vi "Sample mono.vi"() -> ()   [LabVIEW 2018]
uses:
  <vilib>/Instr/_visa.llb/VISA Configure Serial Port (Instr).vi
panel:
  out "output array":i32[](array[numeric])
  in  "array":i32[](array[numeric])=[5, 1, 0, 0]
  out "Set Success":bool
  in  "Value":i32
  out "error out":errorcluster
  out "Comport 2":refnum<visa-resource-name>
  in  "error in (no error)":errorcluster
  in  "Comport":refnum<visa-resource-name>
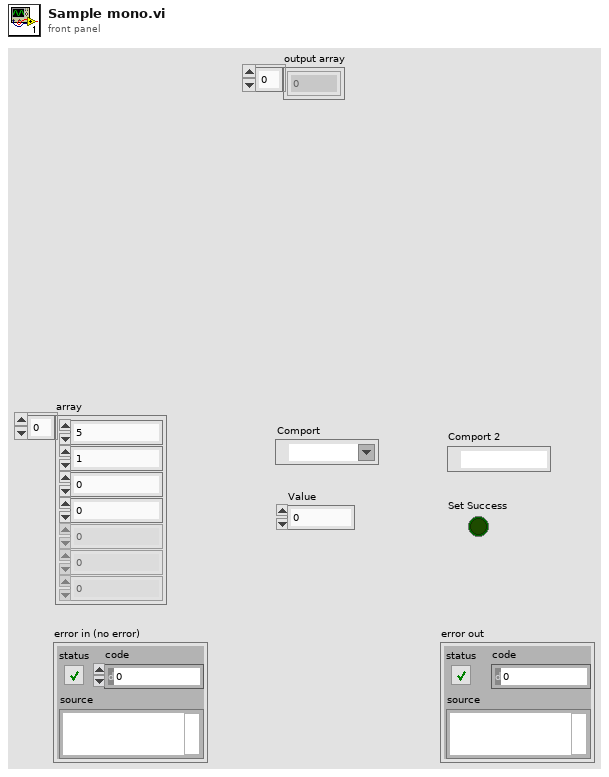
[diagram p1: front panel]
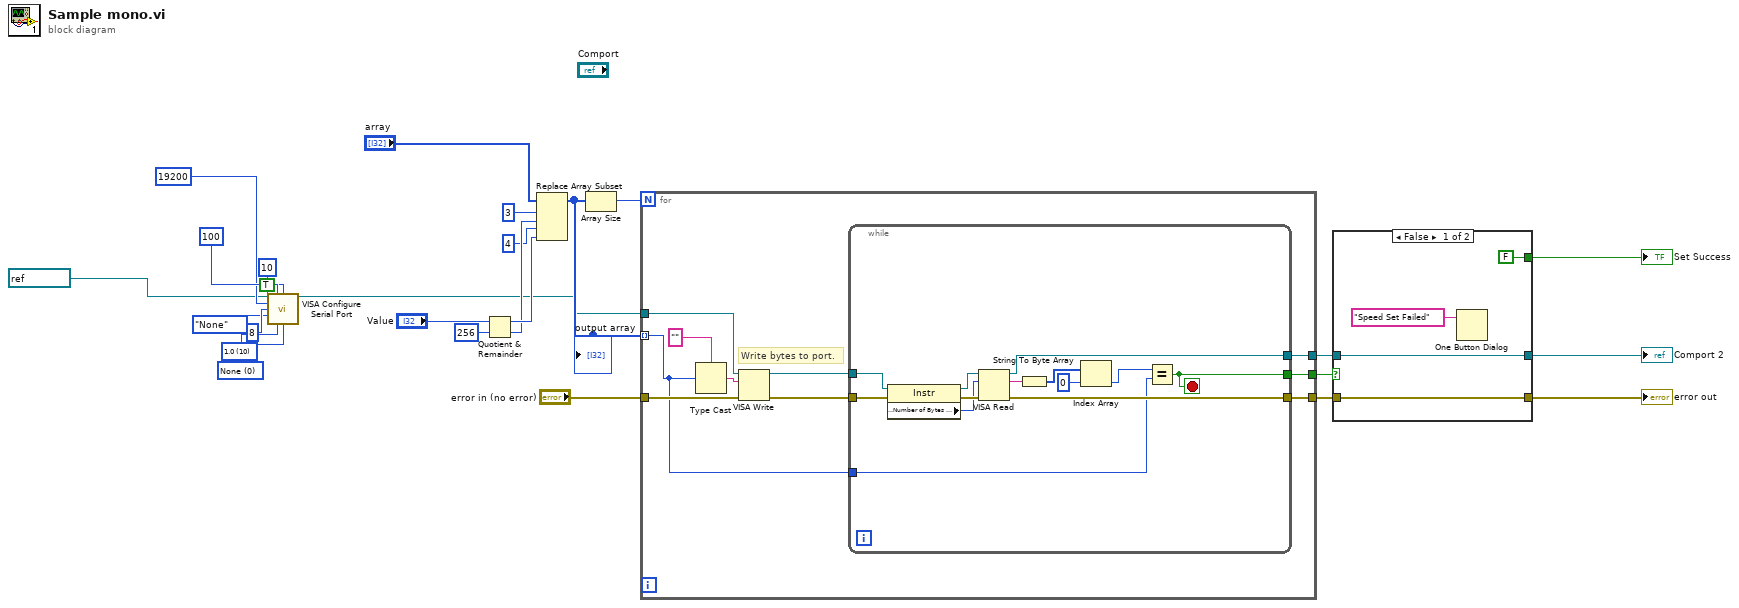
[diagram p0: block diagram]
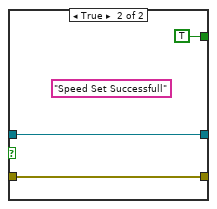
[diagram p2: hidden frame]
diagram:
  w3 = u16 0 items=["None", "XON/XOFF", "RTS/CTS", "XON/XOFF & RTS/CTS", "DTR/DSR", "XON/XOFF & DTR/DSR"] ("flow control (0:none)")
  w4 = u16 10 items=["1.0"=10, "1.5"=15, "2.0"=20] ("stop bits (10: 1 bit)")
  n1 = call-poly "VISA Configure Serial Port"("VISA resource name"=refnum<visa-resource-name> "COM3", "timeout (10sec)"=u32 100, "termination char\n(0xA = '\\n' = LF)"=u8 10 ("termination char\n(0xA = '\\n' = LF)"), "Enable Termination\nChar (T)"=TRUE ("Enable Termination\nChar (T)"), "baud rate (9600)"=u32 19200, "data bits (8)"=u16 8, "parity (0:none)"=enum16{"None", "Odd", "Even", "Mark", "Space"}."None", "stop bits (10: 1 bit)"=w4, "flow control (0:none)"=w3) -> ("VISA resource name out"=w1:refnum<visa-resource-name>)  [unwired: 5 in, 1 out]
  n2 = Quotient & Remainder(x="Value", y=u32 256) -> (x-y*floor(x/y)=w23:u32, floor(x/y)=w22:u32)
  n3 = Replace Array Subset(array="array", new element #1=w22, index #1=3 ("index"), new element #2=w23, index #2=4 ("index")) -> (w20:i32[])
  "output array" <- w20
  n4 = Array Size(array=w20) -> (size(s)=w15:i32)
  n5 = for {
    N: w15 -> [_]
    tunnel: w20 -> [w27] mode=indexing
    tunnel: [w32] -> w16
    tunnel: [w31] -> w14
    tunnel: [w30] -> w13
    tunnel: w1 -> [w29]
    tunnel: "error in (no error)" -> [w28]
    # "Write bytes to port."
    n6 = Type Cast(type="", x=w27) -> (*(type *) &x=w35:string)
    n7 = VISA Write(VISA resource name=w29, write buffer=w35, error in (no error)=w28) -> (VISA resource name out=w34:refnum<visa-resource-name>, error out=w33:errorcluster)  [unwired: 1 out]
    n8 = while {
      tunnel: w34 -> [w42]
      tunnel: w33 -> [w41]
      tunnel: [w45] -> w32
      tunnel: [w44] -> w31
      tunnel: [w43] -> w30
      tunnel: w27 -> [w37]
      stop <- w45 stop-if-true
      n9 = property class="Instr"(reference=w42, error in=w41) -> (reference out=w40:refnum<visa-resource-name>, error out=w39:errorcluster, "Serial Settings:Number of Bytes at Serial Port"=w38:u32)
      n10 = VISA Read(VISA resource name=w40, byte count=w38, error in (no error)=w39) -> (VISA resource name out=w44:refnum<visa-resource-name>, read buffer=w49:string, error out=w43:errorcluster)  [unwired: 1 out]
      n11 = String To Byte Array(string=w49) -> (unsigned byte array=w48:u8[])
      n12 = Index Array(array=w48, index=0) -> (element=w46:u8)
      n13 = Equal?(x=w46, y=w37) -> (x = y?=w45:bool)
    }
  }
  n14 = case shown="False" w16 {
    tunnel: [FALSE TRUE] -> w17
    tunnel: w14 -> [w51 w55]
    tunnel: w13 -> [w50 w54]
    tunnel: [w51 w55] -> w25
    tunnel: [w50 w54] -> w24
    frame False {
      n15 = One Button Dialog(message="Speed Set Failed") -> ()  [unwired: 1 in, 1 out]
    }
    frame True {
      (unwired) "Speed Set Successfull" ("message")
    }
  }
  "Comport 2" <- w25
  "error out" <- w24
  "Set Success" <- w17
